vi "fgv_ctrl-ref.vi"(7 "cmd":enum16{"ini", "read", "write"}(ring), 11 "ref_ctrl_in":T1) -> (3 "ref_ctrl_out":T1)   [LabVIEW 2018]
uses:
  ctrl/control.ctl
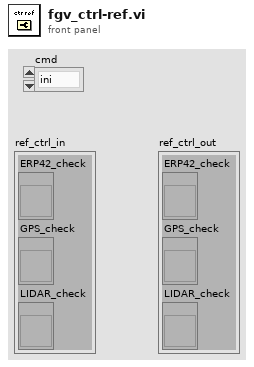
[diagram p1: front panel]
types:
  T1 = typedef "control.ctl" = cluster{"ERP42_check":refnum<vi>, "GPS_check":refnum<vi>, "LIDAR_check":refnum<vi>}
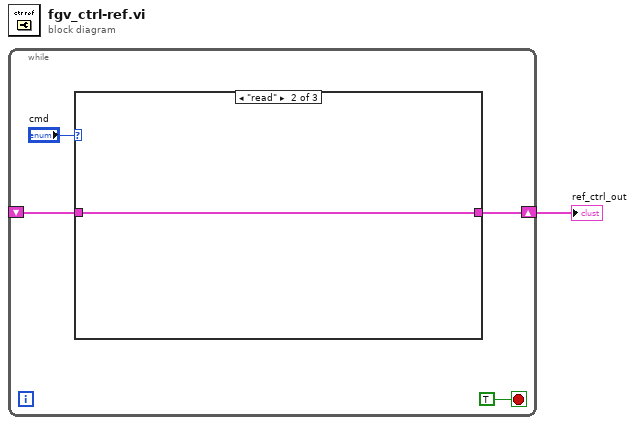
[diagram p0: block diagram]
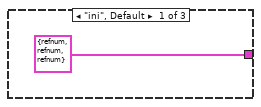
[diagram p2: hidden frame]
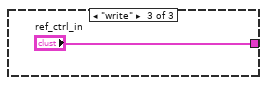
[diagram p3: hidden frame]
diagram:
  n1 = while {
    shift-right: [w3] -> w1
    shift-left: _ -> [w2]
    stop <- TRUE stop-if-true
    n2 = case shown="\"read\"" "cmd" {
      tunnel: [T1 {"ERP42_check"=refnum, "GPS_check"=refnum, "LIDAR_check"=refnum} ("ref_ctrl") w7 "ref_ctrl_in"] -> w3
      tunnel: w2 -> [_ w7 _]
      frame "ini", Default {
      }
      frame "read" {
      }
      frame "write" {
      }
    }
  }
  "ref_ctrl_out" <- w1
